vi "WebSocket_Polling.vi"(8 "error in":errorcluster, 10 "WebSocket Connection":refnum<class "WebSocket Server.lvclass">, 11 "simple_html_chat_ui in":refnum<class "simple_html_chat_ui.lvclass">) -> (0 "error out":errorcluster, 3 "simple_html_chat_ui out":refnum<class "simple_html_chat_ui.lvclass">)   [LabVIEW 2020, in "simple_html_chat_ui.lvclass"]
uses:
  simple_html_chat_ui.lvclass
  WebSockets-API/Source/WebSockets/WebSocket Server/WebSocket Server.lvclass
  typedefs/ui_user_event.ctl
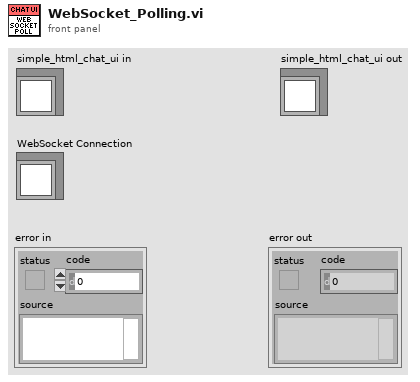
[diagram p1: front panel]
types:
  T1 = typedef "simple_html_chat_ui.lvclass/ui_user_event.ctl" = enum16{"Initialize", "Generate", "Get Reference", "Destroy"}
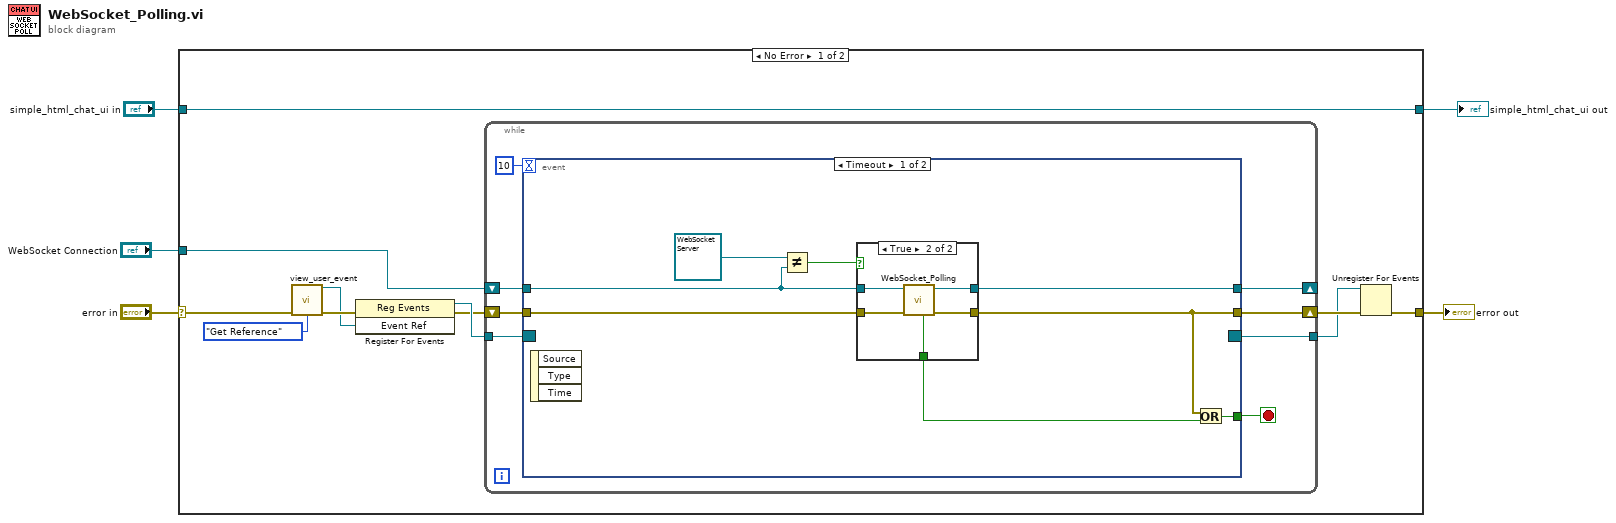
[diagram p0: block diagram]
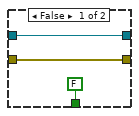
[diagram p2: hidden frame]
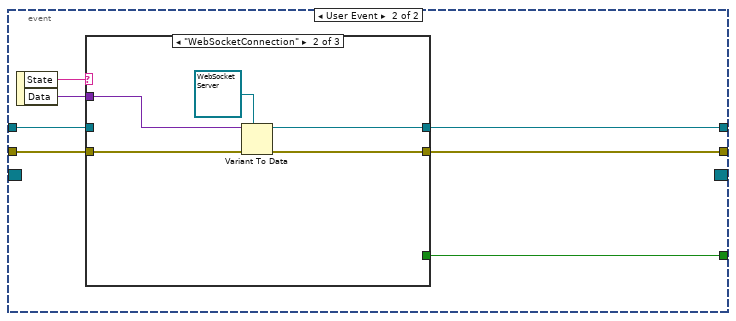
[diagram p3: hidden frame]
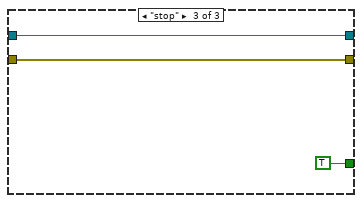
[diagram p5: hidden frame]
diagram:
  n1 = case shown="No Error" "error in" {
    selector: "error in" -> [w7 w58]
    tunnel: "WebSocket Connection" -> [w9 _]
    tunnel: [w8 w58] -> w4
    tunnel: [w6 w59] -> w2
    tunnel: "simple_html_chat_ui in" -> [w6 w59]
    frame No Error {
      n2 = call "view_user_event.vi"("error in (no error)"=w7, "Operation"=ui_user_event."Get Reference") -> ("Event Ref"=w14:refnum<user-event>, "error out"=w15:errorcluster)  [unwired: 12 in]
      n3 = register-events(error in=w15, w14) -> (reference out=w13:refnum<event-registration>, error out=w10:errorcluster)  [unwired: 1 in]
      n4 = while {
        shift-right: [w22] -> w12
        shift-left: w10 -> [w23]
        tunnel: w13 -> [w24]
        tunnel: [w20] -> w11
        shift-right: [w18] -> _
        shift-left: w9 -> [w19]
        stop <- w21 stop-if-true
        n5 = event shown="[0] Timeout" {
          selector: w24 -> [_ _]
          dyn-events: [_ _] -> w20
          timeout: 10 -> [_ _]
          tunnel: w23 -> [w31 w46]
          tunnel: [w29 w44] -> w22
          tunnel: [w32 w43] -> w21
          tunnel: w19 -> [w26 w41]
          tunnel: [w30 w42] -> w18
          event Timeout {
            n6 = event-data() -> ()  [unwired: 1 in, 3 out]
            n7 = Not Equal?(x=refnum<class "WebSocket Server.lvclass"> refnum ("WebSocket Connection"), y=w26) -> (x != y?=w25:bool)
            n8 = case shown="True" w25 {
              tunnel: w31 -> [w35 w40]
              tunnel: w26 -> [w34 w39]
              tunnel: [w34 w38] -> w30
              tunnel: [w35 w37] -> w29
              tunnel: [FALSE ("Boolean") w36] -> w28
              frame False {
              }
              frame True {
                n9 = call "WebSocket_Polling.vi"("error in"=w40, "WebSocket Connection in"=w39) -> ("error out"=w37:errorcluster, "WebSocket Connection out"=w38:refnum<class "WebSocket Server.lvclass">, "Boolean"=w36:bool)  [unwired: 7 in]
              }
            }
            n10 = Or(x=w29, y=w28) -> (x .or. y?=w32:bool)
          }
          event User Event {
            n11 = event-data() -> ("State"=w47:string, "Data"=w45:variant)  [unwired: 1 in]
            n12 = case shown="\"WebSocketConnection\"" w47 {
              tunnel: w46 -> [w49 w54 w57]
              tunnel: w45 -> [_ w52 _]
              tunnel: [w49 w53 w57] -> w44
              tunnel: [_ _ TRUE] -> w43
              tunnel: [w48 w51 w55] -> w42
              tunnel: w41 -> [w48 _ w55]
              frame Default {
              }
              frame "WebSocketConnection" {
                n13 = Variant To Data(error in=w54, type=refnum<class "WebSocket Server.lvclass"> refnum ("WebSocket Connection"), Variant=w52) -> (data=w51:refnum<class "WebSocket Server.lvclass">, error out=w53:errorcluster)
              }
              frame "stop" {
              }
            }
          }
        }
      }
      n14 = Unregister For Events(event registration refnum=w11, error in=w12) -> (error out=w8:errorcluster)
    }
    frame Error {
    }
  }
  "error out" <- w4
  "simple_html_chat_ui out" <- w2
